vi "Generate One Sample.vi"(8 "error in (no error)":errorcluster, 10 "Active channel index":i32, 11 "Channel Settings":T1) -> (0 "error out":errorcluster, 2 "Waveform":waveform(dbl))   [LabVIEW 2021, in "Acquisition.lvlib"]
doc: "Generate one sample for the channel at the 'Active channel index' in the 'Channel Settings' array."
uses:
  Acquisition.lvlib
  Channel Settings.ctl
  IO Device.ctl
  Sensor Type.ctl
  Interval Timer/Interval Timer.lvlib
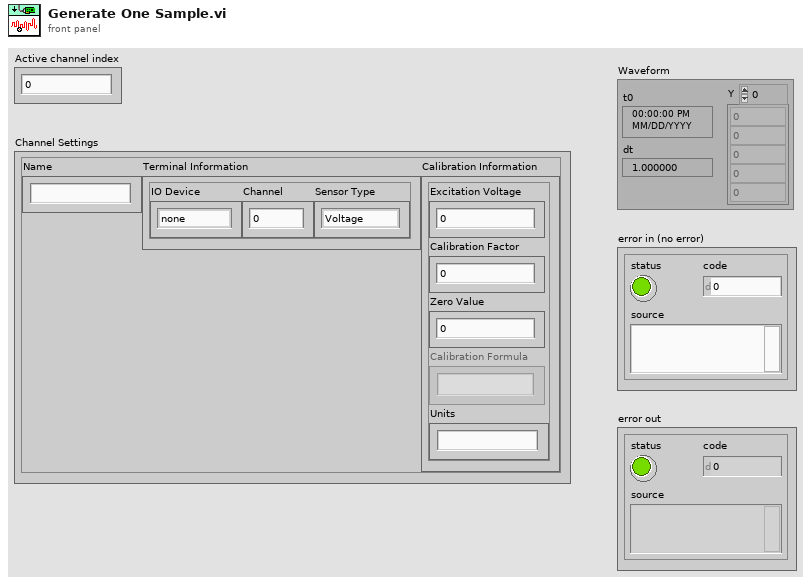
[diagram p1: front panel]
types:
  T1 = typedef "Acquisition.lvlib/Channel Settings.ctl" = cluster{"Name":string, "Terminal Information":cluster{"IO Device":T2, "Channel":i32, "Sensor Type":T3}, "Calibration Information":cluster{"Excitation Voltage":dbl, "Calibration Factor":dbl, "Zero Value":dbl, "Calibration Formula":string, "Units":string}}
  T2 = typedef "Acquisition.lvlib/IO Device.ctl" = enum16{"none", "9219", "9401"}
  T3 = typedef "Acquisition.lvlib/Sensor Type.ctl" = enum16{"Voltage", "Load", "Pressure", "Encoder"}
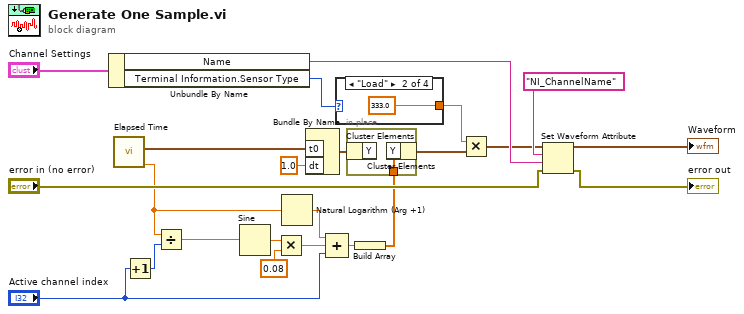
[diagram p0: block diagram]
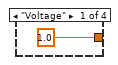
[diagram p2: hidden frame]
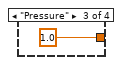
[diagram p3: hidden frame]
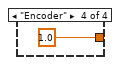
[diagram p4: hidden frame]
diagram:
  n1 = Unbundle By Name("Channel Settings") -> ("Name"=w8:string, "Terminal Information.Sensor Type"=w3:T3)
  n2 = call "Elapsed Time.vi"() -> ("elapsed time (s)"=w19:dbl, "current time"=w10:timestamp)  [unwired: 9 in, 1 out]
  n3 = Increment(x="Active channel index") -> (x+1=w17:i32)
  n4 = Divide(x=w19, y=w17) -> (x/y=w18:dbl)
  n5 = Sine(x=w18) -> (sin(x)=w16:dbl)
  n6 = Multiply(x=w16, y=0.08) -> (x*y=w21:dbl)
  n7 = Natural Logarithm (Arg +1)(1:w19) -> (0:w22:dbl)
  n8 = Bundle By Name("t0"=w10, "dt"=1.0) -> (w13:waveform(dbl))  [unwired: 1 in]
  n9 = Compound Arithmetic op=ADD(w22, w21, "Active channel index") -> (w9:dbl)
  n10 = case shown="\"Load\"" w3 {
    tunnel: [1.0 ("x") 333.0 ("x") 1.0 ("x") 1.0 ("x")] -> w1
    frame "Voltage" {
    }
    frame "Load" {
    }
    frame "Pressure" {
    }
    frame "Encoder" {
    }
  }
  n11 = Build Array(w9) -> (w12:dbl[])
  n12 = in-place {
    in-place-border: w12 -> [w28]
    n13 = in-place-cluster #1(w13) -> ()  [unwired: 1 out]
    n14 = in-place-cluster #1("Y"=w28) -> (w14:waveform(dbl))
  }
  n15 = Multiply(x=w1, y=w14) -> (x*y=w2:waveform(dbl))
  n16 = Set Waveform Attribute(4:"error in (no error)", 5:w8, 6:"NI_ChannelName" ("name"), 7:w2) -> (0:→"error out":errorcluster, 3:→"Waveform":waveform(dbl))  [unwired: 1 out]
